vi "SUB.vi"(4 "Interferent 2:":refnum<vi>, 5 "Komponente:":refnum<vi>, 6 "Interferent 3:":refnum<vi>, 7 "Ring Referenz":refnum<vi>, 8 "Ring Referenz 4":refnum<vi>, 9 "Ring Referenz 3":refnum<vi>, 10 "Ring Referenz 2":refnum<vi>, 11 "Ring (Eingang)":refnum<vi>) -> ()   [LabVIEW 2020]
uses:
  Seiten/FT-IR/FGV FT-IR Gasliste Aktionen.ctl
  Aktion Index uebersetzten.ctl
  Aktion FGV Interference.ctl
  Seiten/FT-IR/FT-IR.lvlib
  Interference verificaton 1065-366.lvlib
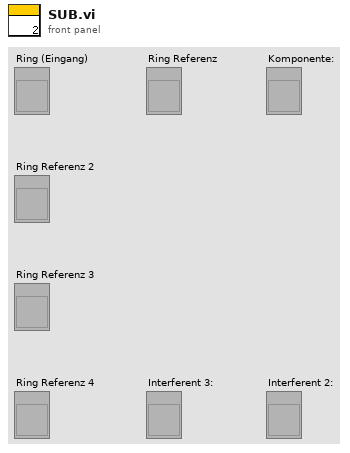
[diagram p1: front panel]
types:
  T1 = typedef "Aktion Index uebersetzten.ctl" = enum16{"lesen", "schreiben", "auswerten"}
  T2 = typedef "FT-IR.lvlib/FGV FT-IR Gasliste Aktionen.ctl" = enum16{"lesen", "Gasliste FT-IR", "Gasliste ausgelesen", "laden", "speichern", "löschen"}
  T3 = typedef "String - Ausgabefeld.ctl" = string
  T4 = typedef "EPA 1065.lvlib/Interference verificaton 1065-366.lvlib/Aktion FGV Interference.ctl" = enum16{"Lesen", "TestKonfig", "Einheiten", "Ergebnis", "Ini", "Tabelle"}
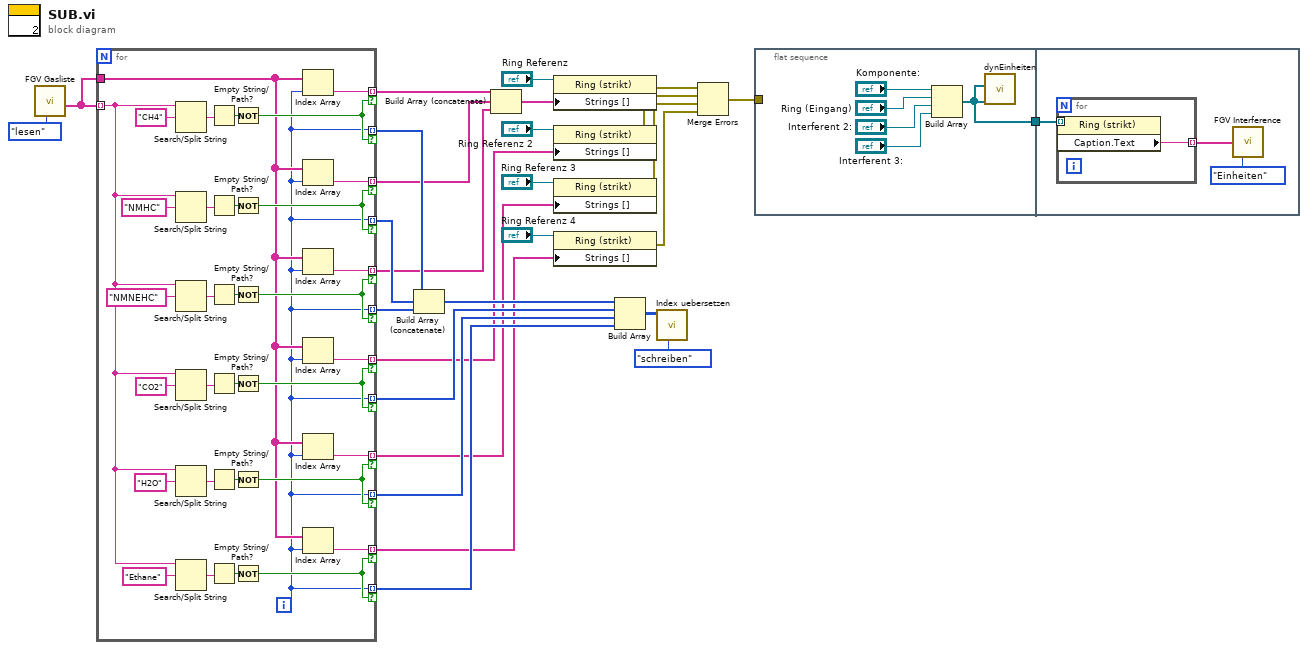
[diagram p0: block diagram]
diagram:
  n1 = call "FGV Gasliste.vi"("Aktionen"=FGV_FT-IR_Gasliste_Aktionen."lesen") -> ("Aktuelle Gasliste gesamt"=w11:T3[])  [unwired: 8 in, 2 out]
  n2 = for {
    tunnel: w11 -> [w31] mode=indexing
    tunnel: w11 -> [w30]
    tunnel: [w58] -> w12 mode=indexing if=w57
    tunnel: [w29] -> w19 mode=indexing if=w57
    tunnel: [w55] -> w13 mode=indexing if=w56
    tunnel: [w29] -> w20 mode=indexing if=w56
    tunnel: [w48] -> w14 mode=indexing if=w47
    tunnel: [w29] -> w21 mode=indexing if=w47
    tunnel: [w45] -> w16 mode=indexing if=w46
    tunnel: [w29] -> w23 mode=indexing if=w46
    tunnel: [w38] -> w17 mode=indexing if=w37
    tunnel: [w29] -> w24 mode=indexing if=w37
    tunnel: [w35] -> w18 mode=indexing if=w36
    tunnel: [w29] -> w25 mode=indexing if=w36
    i -> [w29]
    n3 = Search/Split String(string=w31, search string/char (-)="CH4" ("Such-String/-Zeichen (-)")) -> (match + rest of string=w60:T3)  [unwired: 1 in, 2 out]
    n4 = Search/Split String(string=w31, search string/char (-)="NMHC" ("Such-String/-Zeichen (-)")) -> (match + rest of string=w53:T3)  [unwired: 1 in, 2 out]
    n5 = Search/Split String(string=w31, search string/char (-)="NMNEHC" ("Such-String/-Zeichen (-)")) -> (match + rest of string=w50:T3)  [unwired: 1 in, 2 out]
    n6 = Search/Split String(string=w31, search string/char (-)="CO2" ("Such-String/-Zeichen (-)")) -> (match + rest of string=w43:T3)  [unwired: 1 in, 2 out]
    n7 = Search/Split String(string=w31, search string/char (-)="H2O" ("Such-String/-Zeichen (-)")) -> (match + rest of string=w40:T3)  [unwired: 1 in, 2 out]
    n8 = Search/Split String(string=w31, search string/char (-)="Ethane" ("Such-String/-Zeichen (-)")) -> (match + rest of string=w33:T3)  [unwired: 1 in, 2 out]
    n9 = Empty String/Path?(string/path=w60) -> (empty?=w61:bool)
    n10 = Empty String/Path?(string/path=w53) -> (empty?=w52:bool)
    n11 = Empty String/Path?(string/path=w50) -> (empty?=w51:bool)
    n12 = Empty String/Path?(string/path=w43) -> (empty?=w42:bool)
    n13 = Empty String/Path?(string/path=w40) -> (empty?=w41:bool)
    n14 = Empty String/Path?(string/path=w33) -> (empty?=w32:bool)
    n15 = Not(x=w61) -> (.not. x?=w57:bool)
    n16 = Not(x=w52) -> (.not. x?=w56:bool)
    n17 = Not(x=w51) -> (.not. x?=w47:bool)
    n18 = Not(x=w42) -> (.not. x?=w46:bool)
    n19 = Not(x=w41) -> (.not. x?=w37:bool)
    n20 = Not(x=w32) -> (.not. x?=w36:bool)
    n21 = Index Array(array=w30, index=w29) -> (element=w58:T3)
    n22 = Index Array(array=w30, index=w29) -> (element=w55:T3)
    n23 = Index Array(array=w30, index=w29) -> (element=w48:T3)
    n24 = Index Array(array=w30, index=w29) -> (element=w45:T3)
    n25 = Index Array(array=w30, index=w29) -> (element=w38:T3)
    n26 = Index Array(array=w30, index=w29) -> (element=w35:T3)
  }
  n27 = Build Array (concatenate)(w19, w20, w21) -> (w22:i32[])
  n28 = Build Array (concatenate)(w12, w13, w14) -> (w15:T3[])
  n29 = property on="Eigenschaftsknoten" class="Ring (strikt)"(reference="Ring Referenz", "Strings []"=w15) -> (error out=w6:errorcluster)  [unwired: 1 in, 1 out]
  n30 = property on="Eigenschaftsknoten" class="Ring (strikt)"(reference="Ring Referenz 2", "Strings []"=w16) -> (error out=w7:errorcluster)  [unwired: 1 in, 1 out]
  n31 = property on="Eigenschaftsknoten" class="Ring (strikt)"(reference="Ring Referenz 3", "Strings []"=w17) -> (error out=w8:errorcluster)  [unwired: 1 in, 1 out]
  n32 = property on="Eigenschaftsknoten" class="Ring (strikt)"(reference="Ring Referenz 4", "Strings []"=w18) -> (error out=w9:errorcluster)  [unwired: 1 in, 1 out]
  n33 = Build Array(w22, w23, w24, w25) -> (w26:i32[][])
  n34 = call "Index uebersetzen.vi"("Aktion"=Aktion_Index_uebersetzten."schreiben", "Array"=w26) -> ()  [unwired: 8 in, 2 out]
  n35 = Merge Errors(w6, w7, w8, w9) -> (w10:errorcluster)
  n36 = flat-sequence {
    tunnel: w10 -> [_]
    tunnel: [w62] -> w28
    tunnel: w28 -> [w69]
    frame #0 {
      n37 = Build Array("Komponente:", "Ring (Eingang)", "Interferent 2:", "Interferent 3:") -> (w62:refnum<vi>[])
      n38 = call "dynEinheiten.vi"("Komponenten Ref."=w62, "Sollwert Ref."=w62) -> ()  [unwired: 10 in]
    }
    frame #1 {
      n39 = for {
        tunnel: w69 -> [w71] mode=indexing
        tunnel: [w70] -> w67 mode=indexing
        n40 = property class="Ring (strikt)"(reference=w71) -> ("Caption.Text"=w70:string)  [unwired: 1 in, 2 out]
      }
      n41 = call "FGV Interference.vi"("Êinheiten"=w67, "Aktion FGV Interference"=Aktion_FGV_Interference."Einheiten") -> ()  [unwired: 9 in, 5 out]
    }
  }
